vi "NI VeriStand - Register Custom Device Engine Events.vi"(8 "error in (no error)":errorcluster, 11 "Device Ref in":T2 format="%.0x") -> (0 "error out":errorcluster, 2 "Custom Device Engine Event Ref":T1, 3 "Device Ref out":T2 format="%.0x")   [LabVIEW 2020, in "Custom Device API.lvlib"]
doc: "Dynamically registers custom device engine events. This VI registers the events Shut Down, Message (Byte Array), and Message (String). The Shut Down event is triggered when the custom device engine shuts down. The Message events trigger when the NI VeriStand - Send Custom Device Message VI or a corresponding .NET method is called."
uses:
  <vilib>/NI VeriStand/Custom Device API/Custom Device API.lvlib
  <vilib>/NI VeriStand/Custom Device API/Custom Device Item Ref.ctl
  <vilib>/NI VeriStand/Custom Device API/Custom Device Engine Event Ref.ctl
  <vilib>/NI VeriStand/Custom Device API/Custom Device Communication Bus.ctl
  <vilib>/NI VeriStand/Custom Device API/Message (String).ctl
  <vilib>/NI VeriStand/Custom Device API/Message Response (String).ctl
  <vilib>/NI VeriStand/Custom Device API/Message (Byte Array).ctl
  <vilib>/NI VeriStand/Custom Device API/Message Response (Byte Array).ctl
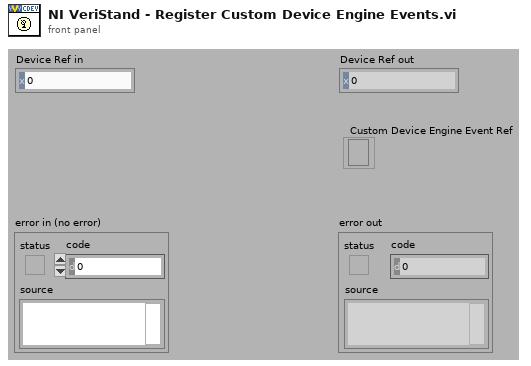
[diagram p1: front panel]
types:
  T1 = typedef "Custom Device API.lvlib/Custom Device Engine Event Ref.ctl" = refnum<event-registration>
  T2 = typedef "Custom Device API.lvlib/Custom Device Item Ref.ctl" = u64
  T3 = typedef "Custom Device API.lvlib/Custom Device Communication Bus.ctl" = cluster{"Message (String)":refnum<user-event>, "Message (Byte Array)":refnum<user-event>, "Shut Down":refnum<user-event>, "Event Ref":T1}
  T4 = typedef "Custom Device API.lvlib/Message (Byte Array).ctl" = cluster{"Command":string, "Data":u8[], "Response Event":refnum<user-event>}
  T5 = typedef "Custom Device API.lvlib/Message (String).ctl" = cluster{"Command":string, "Data":string, "Response Event":refnum<user-event>}
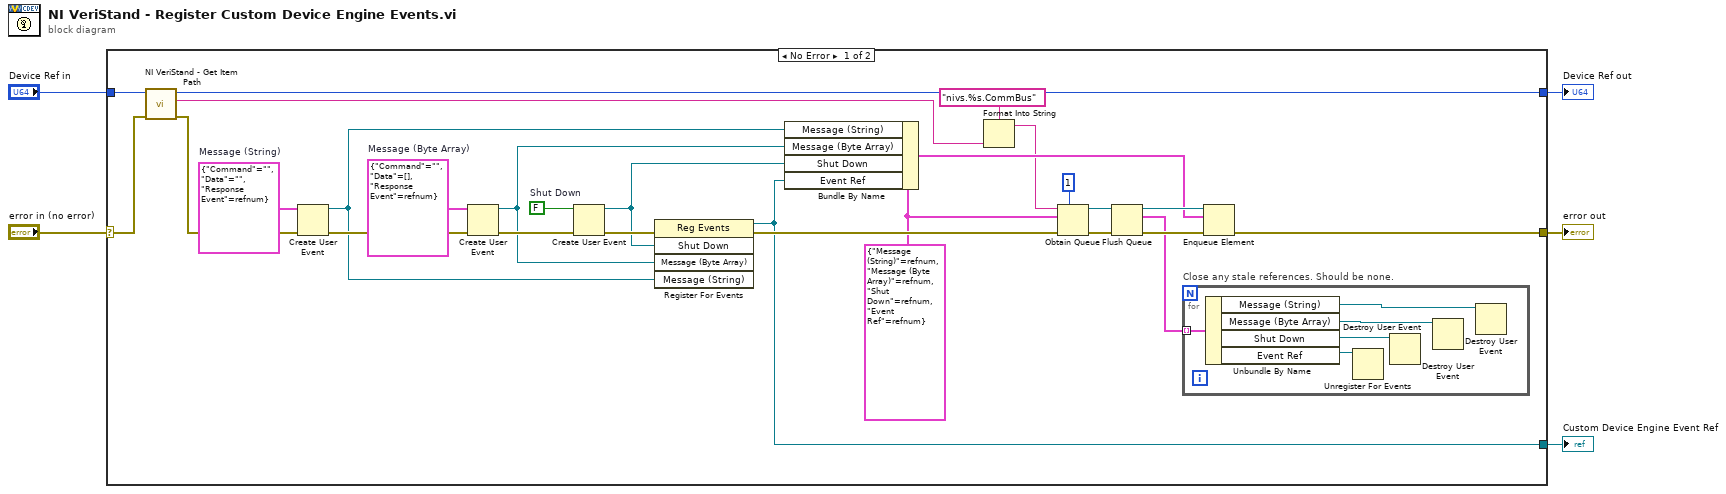
[diagram p0: block diagram]
diagram:
  n1 = case shown="No Error" "error in (no error)" {
    selector: "error in (no error)" -> [w28 w38]
    tunnel: [w23 w39] -> w4
    tunnel: "Device Ref in" -> [w29 w39]
    tunnel: [w11 w38] -> w2
    tunnel: [w9 _] -> w1
    frame No Error {
      w16 = T3 {"Message (String)"=refnum, "Message (Byte Array)"=refnum, "Shut Down"=refnum, "Event Ref"=refnum} ("Communication Bus")
      w25 = FALSE  # Shut Down
      w26 = T4 {"Command"="", "Data"=[], "Response Event"=refnum}  # Message (Byte Array)
      w27 = T5 {"Command"="", "Data"="", "Response Event"=refnum}  # Message (String)
      n2 = call <vilib>:"NI VeriStand - Get Item Path.vi"("error in (no error)"=w28, "Item Ref in"=w29) -> ("error out"=w24:errorcluster, "Path"=w7:string, "Item Ref out"=w23:T2)  [unwired: 6 in, 1 out]
      n3 = Create User Event(user event datatype=w27, error in=w24) -> (user event=w19:refnum<user-event>, error out=w22:errorcluster)
      n4 = Create User Event(user event datatype=w26, error in=w22) -> (user event=w18:refnum<user-event>, error out=w21:errorcluster)
      n5 = Create User Event(user event datatype=w25, error in=w21) -> (user event=w17:refnum<user-event>, error out=w20:errorcluster)
      n6 = register-events(error in=w20, w17, w18, w19) -> (reference out=w9:refnum<event-registration>, error out=w31:errorcluster)  [unwired: 1 in]
      n7 = Bundle By Name(cluster=w16, "Message (String)"=w19, "Message (Byte Array)"=w18, "Shut Down"=w17, "Event Ref"=w9) -> (w30:T3)
      n8 = Format Into String(format string="nivs.%s.CommBus", w7) -> (resulting string=w6:string)  [unwired: 2 in, 1 out]
      n9 = Obtain Queue(max queue size (-1, unlimited)=1, name (unnamed)=w6, element data type=w16, error in (no error)=w31) -> (queue out=w15:refnum<queue>, error out=w14:errorcluster)  [unwired: 1 in, 1 out]
      n10 = Flush Queue(queue=w15, error in (no error)=w14) -> (queue out=w32:refnum<queue>, remaining elements=w10:T3[], error out=w12:errorcluster)
      n11 = for "Close any stale references. Should be none." {
        tunnel: w10 -> [w37] mode=indexing
        n12 = Unbundle By Name(w37) -> ("Message (String)"=w33:refnum<user-event>, "Message (Byte Array)"=w34:refnum<user-event>, "Shut Down"=w35:refnum<user-event>, "Event Ref"=w36:T1)
        n13 = Unregister For Events(event registration refnum=w36) -> ()  [unwired: 1 in, 1 out]
        n14 = Destroy User Event(user event=w35) -> ()  [unwired: 1 in, 1 out]
        n15 = Destroy User Event(user event=w34) -> ()  [unwired: 1 in, 1 out]
        n16 = Destroy User Event(user event=w33) -> ()  [unwired: 1 in, 1 out]
      }
      n17 = Enqueue Element(queue=w32, element=w30, error in (no error)=w12) -> (error out=w11:errorcluster)  [unwired: 1 in, 2 out]
    }
    frame Error {
    }
  }
  "Device Ref out" <- w4
  "error out" <- w2
  "Custom Device Engine Event Ref" <- w1
